vi "latch.vi"(10 "InControl":bool) -> (2 "Boolean":bool)   [LabVIEW 2014]
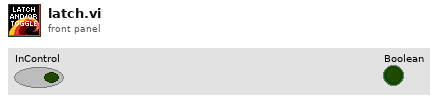
[diagram p1: front panel]
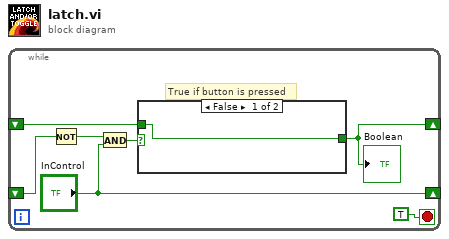
[diagram p0: block diagram]
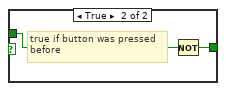
[diagram p2: hidden frame]
diagram:
  n1 = while {
    shift-right: [w7] -> _
    shift-left: _ -> [w6]
    shift-right: ["InControl"] -> _
    shift-left: _ -> [w2]
    stop <- TRUE stop-if-true
    # "True if button is pressed"
    n2 = Not(x=w2) -> (.not. x?=w4:bool)
    n3 = And(x=w4, y="InControl") -> (x .and. y?=w3:bool)
    n4 = case shown="False" w3 {
      tunnel: [w8 w10] -> w7
      tunnel: w6 -> [w8 w9]
      frame False {
      }
      frame True {
        # "true if button was pressed\nbefore"
        n5 = Not(x=w9) -> (.not. x?=w10:bool)
      }
    }
    "Boolean" <- w7
  }
